vi "Splice Periodic Waveform.vi"(8 "Error In":errorcluster, 10 "Y Array":dbl[](array[numeric]), 11 "X Array":dbl[](array[numeric])) -> (0 "Error Out":errorcluster, 3 "Output arrays":cluster{"Array":dbl[], "Array":dbl[]}[](array[cluster]))   [LabVIEW 2016]
uses:
  <vilib>/measure/matone.llb/Extract Single Tone Information 1 Chan.vi
  <vilib>/measure/NI_MAPro.lvlib
  <vilib>/Analysis/NI_AAL_SigProc.lvlib
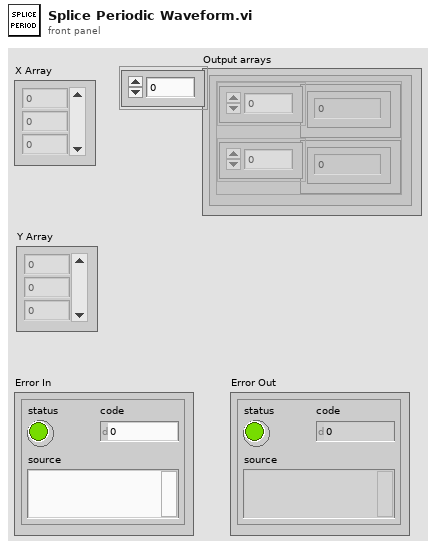
[diagram p1: front panel]
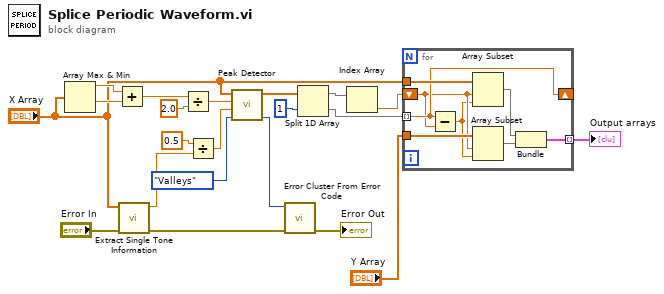
[diagram p0: block diagram]
diagram:
  n1 = Array Max & Min(array="X Array") -> (max value=w21:dbl, min value=w20:dbl)  [unwired: 2 out]
  n2 = Add(x=w21, y=w20) -> (x+y=w19:dbl)
  n3 = call-poly <vilib>:"Extract Single Tone Information.vi"("error in (no error)"="Error In", "time signal in"="X Array") -> ("error out"=w2:errorcluster, "detected frequency"=w14:dbl)  [unwired: 4 in, 4 out]
  n4 = Divide(x=w19, y=2.0) -> (x/y=w17:dbl)
  n5 = Divide(x=0.5, y=w14) -> (x/y=w13:dbl)
  n6 = call <vilib>:"Peak Detector.vi"("peaks/valleys"=enum32{"Peaks", "Valleys"}."Valleys", "width"=w13, "threshold"=w17, "X"="X Array") -> ("error"=w3:i32, "Locations"=w12:dbl[])  [unwired: 3 in, 3 out]
  n7 = call <vilib>:"Error Cluster From Error Code.vi"("error in (no error)"=w2, "error code (0)"=w3) -> ("error out"=→"Error Out":errorcluster)  [unwired: 7 in]
  n8 = Split 1D Array(array=w12, index=1) -> (first subarray=w9:dbl[], second subarray=w10:dbl[])
  n9 = Index Array(array=w9) -> (element=w8:dbl)  [unwired: 1 in]
  n10 = for {
    tunnel: w10 -> [w27] mode=indexing
    tunnel: "X Array" -> [w29]
    tunnel: "Y Array" -> [w28]
    shift-right: [w27] -> _
    shift-left: w8 -> [w26]
    tunnel: [w22] -> w5 mode=indexing
    n11 = Subtract(x=w27, y=w26) -> (x-y=w25:dbl)
    n12 = Array Subset(array=w29, index=w26, length=w25) -> (w24:dbl[])
    n13 = Array Subset(array=w28, index=w26, length=w25) -> (w23:dbl[])
    n14 = Bundle(w24, w23) -> (w22:cluster{dbl[], dbl[]})  [unwired: 1 in]
  }
  "Output arrays" <- w5
